vi "FGV Analysator Definition.vi"(6 "Aktionen":T5, 7 "Analysator Auswahl":T1 {"Analysator Auswahl 12" items=["----"=100, "FT-IR"=0, "TEST"=1]; "Analysator Auswahl 11" items=["----"=100, "FT-IR"=0, "TEST"=1]; "Analysator Auswahl 10" items=["----"=100, "FT-IR"=0, "TEST"=1]; "Analysator Auswahl 9" items=["----"=100, "FT-IR"=0, "TEST"=1]; "Analysator Auswahl 8" items=["----"=100, "FT-IR"=0, "TEST"=1]; "Analysator Auswahl 7" items=["----"=100, "FT-IR"=0, "TEST"=1]; "Analysator Auswahl 6" items=["----"=100, "FT-IR"=0, "TEST"=1]; "Analysator Auswahl 5" items=["----"=100, "FT-IR"=0, "TEST"=1]; "Analysator Auswahl 4" items=["----"=100, "FT-IR"=0, "TEST"=1]; "Analysator Auswahl 3" items=["----"=100, "FT-IR"=0, "TEST"=1]; "Analysator Auswahl 2" items=["----"=100, "FT-IR"=0, "TEST"=1]; "Analysator Auswahl" items=["----"=100, "FT-IR"=0, "PMA"=1]}, 8 "error in (no error)":errorcluster caption="Fehler (Eingang, kein Fehler)", 9 "Messbereiche KAL":T4[](array[typedef]), 10 "Messbereich":i32, 11 "Komponente":i32) -> (0 "error out":errorcluster caption="Fehler (Ausgang)", 1 "Betriebsdaten Komponente":T3, 2 "Betriebsdaten":T3[](array[typedef]), 3 "Analysatoren":string[](array[string]), 5 "max SpanEingang":i32)   [LabVIEW 2020, in "Analysator Definition.lvlib"]
doc: "0...........FTIR\n1...........PMA\n2...........FID CH4\n3...........FID THC\n4...........FID NMHC"
uses:
  Analysator Definition.lvlib
  FGV Analysator Definition Aktionen.ctl
  Betriebsdaten Komponente.ctl
  Visualisierungs Elemente/Auswahlfeld.ctl
  Seiten/CalGas Aufschaltung/Cluster Auswahl Analysator.ctl
  Seiten/CalGas Aufschaltung/Analysator Auswahl.ctl
  Analysator Definition.ctl
  Seiten/CalGas Aufschaltung/CalGas Aufschaltung.lvlib
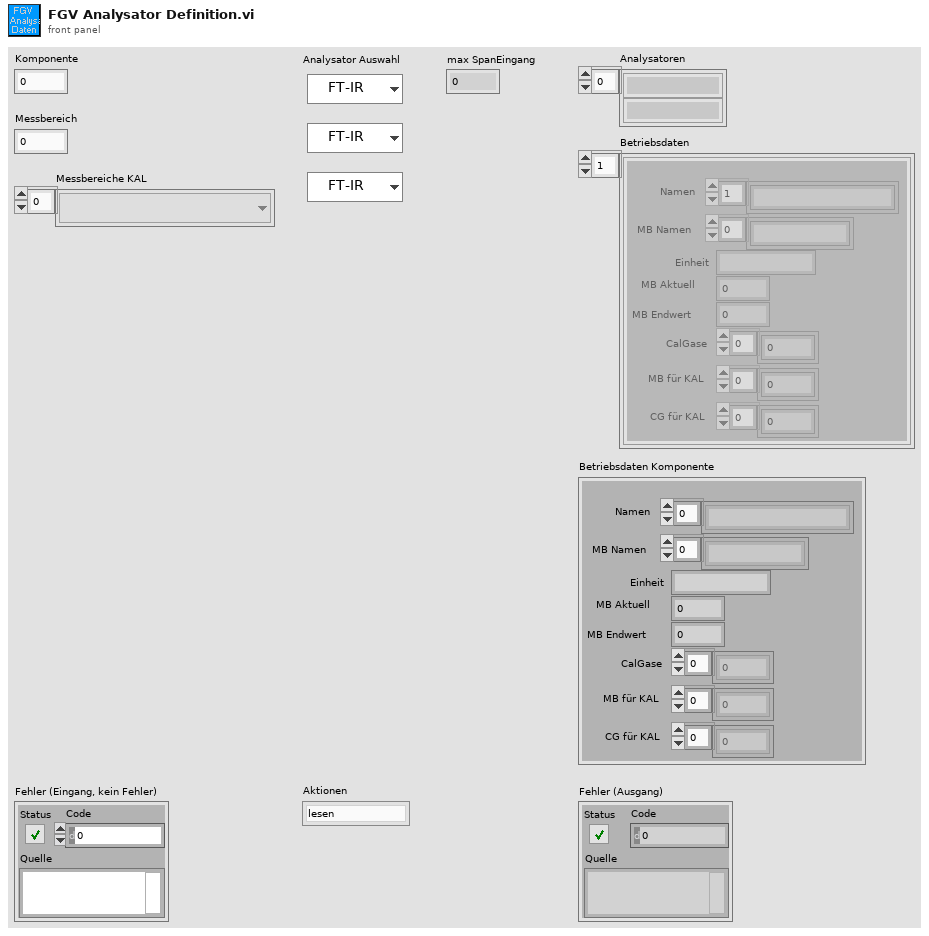
[diagram p1: front panel]
types:
  T1 = typedef "CalGas Aufschaltung.lvlib/Cluster Auswahl Analysator.ctl" = cluster{"Analysator Auswahl":T2, "Analysator Auswahl 2":T2, "Analysator Auswahl 3":T2, "Analysator Auswahl 4":T2, "Analysator Auswahl 5":T2, "Analysator Auswahl 6":T2, "Analysator Auswahl 7":T2, "Analysator Auswahl 8":T2, "Analysator Auswahl 9":T2, "Analysator Auswahl 10":T2, "Analysator Auswahl 11":T2, "Analysator Auswahl 12":T2}
  T2 = typedef "CalGas Aufschaltung.lvlib/Analysator Auswahl.ctl" = u16
  T3 = typedef "Analysator Definition.lvlib/Betriebsdaten Komponente.ctl" = cluster{"Namen":string[], "MB Namen":string[], "Einheit":string, "MB Aktuell":u16, "MB Endwert":u16, "CalGase":u16[], "MB für KAL":u16[], "CG für KAL":u16[]}
  T4 = typedef "Auswahlfeld.ctl" = u16
  T5 = typedef "Analysator Definition.lvlib/FGV Analysator Definition Aktionen.ctl" = enum16{"lesen", "MB setzen", "MB KAL setzen", "laden"}
  T6 = typedef "Analysator Definition.lvlib/Analysator Definition.ctl" = string[][]
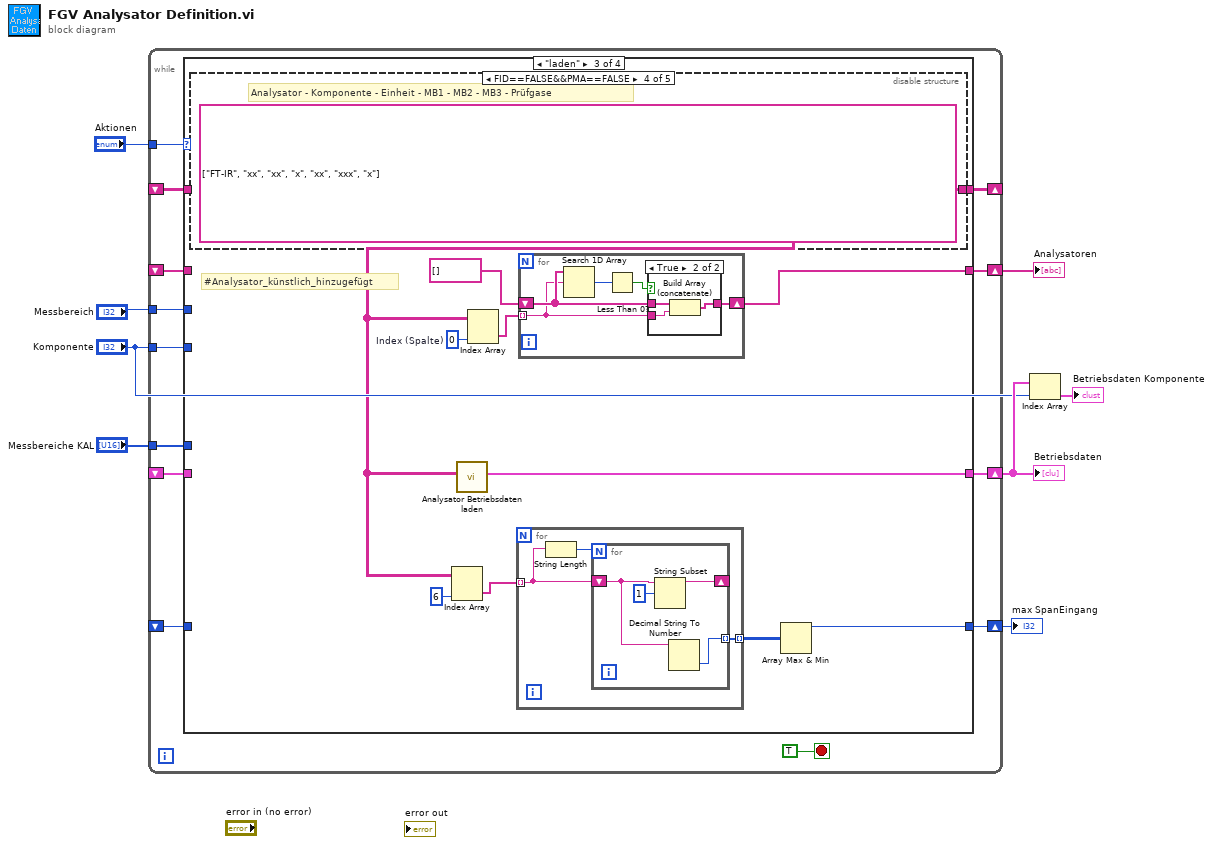
[diagram p0: block diagram]
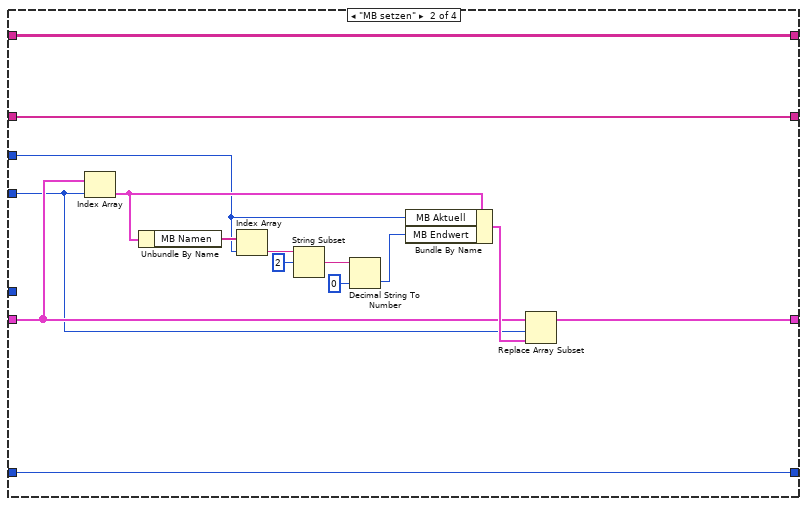
[diagram p3: hidden frame]
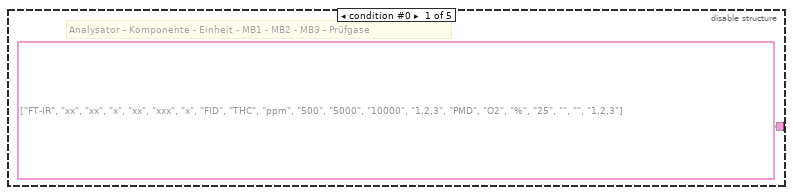
[diagram p4: hidden frame]
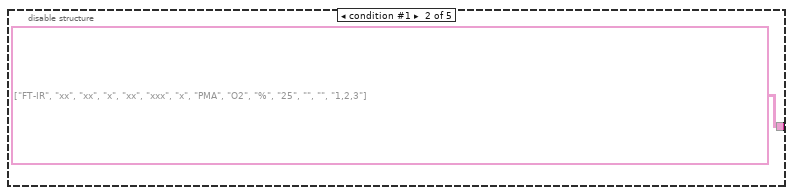
[diagram p5: hidden frame]
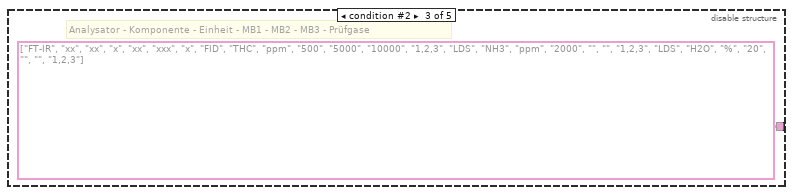
[diagram p6: hidden frame]
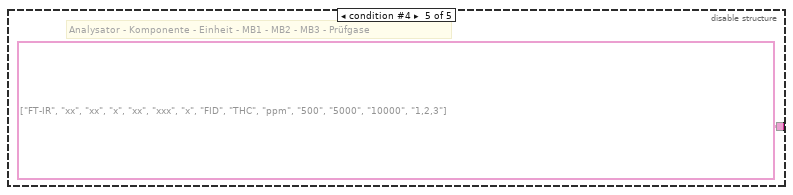
[diagram p7: hidden frame]
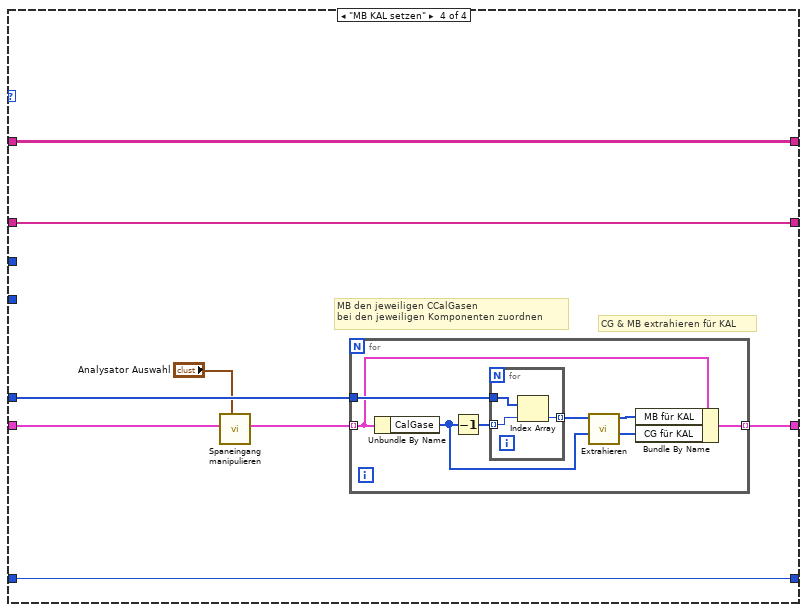
[diagram p9: hidden frame]
diagram:
  n1 = while {
    tunnel: "Aktionen" -> [w20]
    shift-right: [w19] -> _
    shift-left: _ -> [w18]
    shift-right: [w17] -> w7
    shift-left: _ -> [w16]
    shift-right: [w12] -> w4
    shift-left: _ -> [w15]
    tunnel: "Komponente" -> [w11]
    tunnel: "Messbereich" -> [w14]
    tunnel: "Messbereiche KAL" -> [w13]
    shift-right: [w10] -> w1
    shift-left: _ -> [w9]
    stop <- TRUE stop-if-true
    n2 = case shown="\"laden\"" w20 {
      tunnel: [w25 w39 w44 w79] -> w19
      tunnel: w18 -> [w25 w39 _ w79]
      tunnel: [w24 w40 w48 w78] -> w17
      tunnel: w16 -> [w24 w40 _ w78]
      tunnel: [w23 w30 w46 w77] -> w12
      tunnel: w15 -> [w23 w31 _ w74]
      tunnel: w11 -> [_ w28 _ _]
      tunnel: w14 -> [_ w27 _ _]
      tunnel: w13 -> [_ _ _ w76]
      tunnel: [w22 w26 w41 w75] -> w10
      tunnel: w9 -> [w22 w26 _ w75]
      frame "lesen", Default {
      }
      frame "MB setzen" {
        n3 = Index Array(array=w31, index=w28) -> (element=w38:T3)
        n4 = Unbundle By Name(w38) -> ("MB Namen"=w37:string[])
        n5 = Index Array(array=w37, index=w27) -> (element=w36:string)
        n6 = String Subset(string=w36, offset (0)=2 ("Offset (0)")) -> (substring=w33:string)  [unwired: 1 in]
        n7 = Decimal String To Number(string=w33, default (0L)=u16 0 ("Standard (0 I32)")) -> (number=w29:u16)  [unwired: 1 in, 1 out]
        n8 = Bundle By Name(cluster=w38, "MB Aktuell"=w27, "MB Endwert"=w29) -> (w32:T3)
        n9 = Replace Array Subset(array=w31, new element=w32, index=w28) -> (w30:T3[])
      }
      frame "laden" {
        w47 = 0  # Index (Spalte)
        # "#Analysator_künstlich_hinzugefügt"
        n10 = disable-structure shown="FID==FALSE&&PMA==FALSE" {
          disable-tunnel: [T6 [["FT-IR", "xx", "xx", "x", "xx", "xxx", "x"], ["FID", "THC", "ppm", "500", "5000", "10000", "1,2,3"], ["PMD", "O2", "%", "25", "", "", "1,2,3"]] ("Analysator Definition") T6 [["FT-IR", "xx", "xx", "x", "xx", "xxx", "x"], ["PMA", "O2", "%", "25", "", "", "1,2,3"]] ("Analysator Definition") T6 [["FT-IR", "xx", "xx", "x", "xx", "xxx", "x"], ["FID", "THC", "ppm", "500", "5000", "10000", "1,2,3"], ["LDS", "NH3", "ppm", "2000", "", "", "1,2,3"], ["LDS", "H2O", "%", "20", "", "", "1,2,3"]] ("Analysator Definition") T6 [["FT-IR", "xx", "xx", "x", "xx", "xxx", "x"]] ("Analysator Definition") T6 [["FT-IR", "xx", "xx", "x", "xx", "xxx", "x"], ["FID", "THC", "ppm", "500", "5000", "10000", "1,2,3"]] ("Analysator Definition")] -> w44
          frame condition #0 {
            # "Analysator - Komponente - Einheit - MB1 - MB2 - MB3 - Prüfgase"
            # "Analysatoren Filtern"
          }
          frame condition #1 {
          }
          frame condition #2 {
            # "Analysator - Komponente - Einheit - MB1 - MB2 - MB3 - Prüfgase"
            # "Analysatoren Filtern"
          }
          frame condition #3 (active) {
            # "Analysator - Komponente - Einheit - MB1 - MB2 - MB3 - Prüfgase"
            # "Analysatoren Filtern"
          }
          frame condition #4 {
            # "Analysator - Komponente - Einheit - MB1 - MB2 - MB3 - Prüfgase"
            # "Analysatoren Filtern"
          }
        }
        n11 = Index Array(array=w44, index (col)=6 ("Deaktivierter Index (Spalte)")) -> (element=w43:string[])  [unwired: 1 in]
        n12 = call "Analysator Betriebsdaten laden.vi"("Analysator Definition"=w44) -> ("Betriebsdaten"=w46:T3[])  [unwired: 10 in]
        n13 = Index Array(array=w44, index (col)=w47) -> (element=w49:string[])  [unwired: 1 in]
        n14 = for {
          tunnel: w43 -> [w52] mode=indexing
          tunnel: [w51] -> w42 mode=indexing
          n15 = String Length(string=w52) -> (length=w53:i32)
          n16 = for {
            N: w53 -> [_]
            shift-right: [w57] -> _
            shift-left: w52 -> [w55]
            tunnel: [w56] -> w51 mode=indexing
            n17 = String Subset(string=w55, offset (0)=1 ("Offset (0)")) -> (substring=w57:string)  [unwired: 1 in]
            n18 = Decimal String To Number(string=w55) -> (number=w56:i32)  [unwired: 2 in, 1 out]
          }
        }
        n19 = for {
          tunnel: w49 -> [w65] mode=indexing
          shift-right: [w63] -> w48
          shift-left: string[] [] ("Teil-Array") -> [w66]
          n20 = Search 1D Array(1D array=w66, element=w65) -> (index of element=w67:i32)  [unwired: 1 in]
          n21 = Less Than 0?(x=w67) -> (x < 0?=w64:bool)
          n22 = case shown="True" w64 {
            tunnel: w66 -> [w68 w71]
            tunnel: w65 -> [_ w70]
            tunnel: [w68 w69] -> w63
            frame False {
            }
            frame True {
              n23 = Build Array (concatenate)(w71, w70) -> (w69:string[])
            }
          }
        }
        n24 = Array Max & Min(array=w42) -> (max value=w41:i32)  [unwired: 3 out]
      }
      frame "MB KAL setzen" {
        # "CG & MB extrahieren für KAL"
        # "MB den jeweiligen CCalGasen \nbei den jeweiligen Komponenten zuordnen"
        n25 = call "Spaneingang manipulieren.vi"("Analysator Auswahl"="Analysator Auswahl", "Betriebsdaten"=w74) -> ("Betriebsdaten"=w73:T3[])  [unwired: 8 in, 1 out]
        n26 = for {
          tunnel: w73 -> [w80] mode=indexing
          tunnel: w76 -> [w87]
          tunnel: [w81] -> w77 mode=indexing
          n27 = Unbundle By Name(w80) -> ("CalGase"=w85:u16[])
          n28 = Decrement(x=w85) -> (x-1=w84:u16[])
          n29 = for {
            tunnel: w84 -> [w90] mode=indexing
            tunnel: w87 -> [w89]
            tunnel: [w88] -> w86 mode=indexing
            n30 = Index Array(array=w89, index=w90) -> (element=w88:T4)
          }
          n31 = call "Extrahieren.vi"("Cal Gase"=w85, "Messbereiche"=w86) -> ("Cal Gase"=w82:u16[], "Messbereiche"=w83:u16[])  [unwired: 8 in]
          n32 = Bundle By Name(cluster=w80, "MB für KAL"=w83, "CG für KAL"=w82) -> (w81:T3)
        }
      }
    }
  }
  "Analysatoren" <- w7
  "Betriebsdaten" <- w4
  "max SpanEingang" <- w1
  n33 = Index Array(array=w4, index="Komponente") -> (element=→"Betriebsdaten Komponente":T3)
